vi "Get Set Point (SubVI).vi"   [LabVIEW 2014]
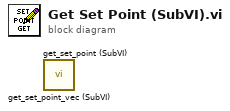
[diagram p0: block diagram]
diagram:
  n1 = call "get_set_point_vec (SubVI).vi"() -> ()  [unwired: 2 in, 2 out]
  n2 = call "get_set_point (SubVI).vi"() -> ()  [unwired: 2 in, 2 out]
